vi "Autonomous Independent.vi"() -> ()   [LabVIEW 2014]
doc: "This VI is called when autonomous begins, and will automatically be terminated when autonomous ends. You can carry out timed or sensor driven robot movement independently without needing to return to the caller."
uses:
  <vilib>/Rock Robotics/WPI/Joystick/WPI_JoystickGetSetRefNum.vi
  <vilib>/Rock Robotics/Network Tables/SD Read Number.vi
  <vilib>/Rock Robotics/Network Tables/SD Write String.vi
  <vilib>/Rock Robotics/WPI/RobotDrive/WPI_RobotDriveGetSetRefNum.vi
  <vilib>/Rock Robotics/WPI/RobotDrive/WPI_RobotDriveArcadeDrive_Standard(NoSaturation).vi
panel:
  out "Current Movement, for debugging":T1 {"Y Joystick Value" scale=1.0..-1.0; "X Joystick Value" scale=-1.0..1.0}
  in  "Array of robot movements":T2(array[cluster]) {"Y Joystick Value" scale=1.0..-1.0; "X Joystick Value" scale=-1.0..1.0}
  # "Be sure to right-click and choose Data Operations>>Make Current Value default if you want to save the array values with the VI"
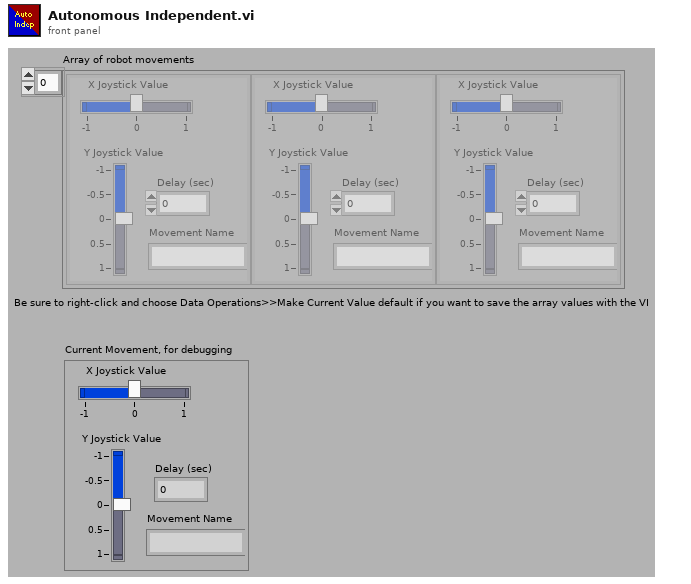
[diagram p1: front panel]
types:
  T1 = cluster{"X Joystick Value":dbl, "Y Joystick Value":dbl, "Delay (sec)":dbl, "Movement Name":string}
  T2 = cluster{"X Joystick Value":dbl, "Y Joystick Value":dbl, "Delay (sec)":dbl, "Movement Name":string}[]
  T3 = typedef "WPI_JoystickDevRef.ctl" = cluster{"Device":T4}
  T4 = typedef "WPI_JoystickDeviceEnum.ctl" = enum16{"USB 0", "USB 1", "USB 2", "USB 3", "USB 4", "USB 5"}
  T5 = typedef "WPI_RobotDriveDevRef.ctl" = cluster{"DevStatus":errorcluster, "Motors[]":T6[], "Square Inputs":bool, "Max Output":dbl}
  T6 = typedef "WPI_MotorControlDeviceRef.ctl" = cluster{"DeviceStatus":errorcluster, "Type":T7, "PWM":cluster{"Controller":T8, "PWM Channel":T9, "DeadBand":T10}, "CAN":cluster{"Device Number":u8, "Control Mode":T11, "Semaphore":T12, "Max Vout":dbl, "TalonSRX Control Mode":T13}, "Invert":bool, "TransformRef":T14, "InvTransformRef":T14}
  T7 = typedef "WPI_MotorControlType.ctl" = enum16{"PWM", "CAN", "CANTalonSRX"}
  T8 = typedef "FPGA_TypedefDigitalModule.ctl" = enum16{"Controller 1"}
  T9 = typedef "FPGA_DIOPWMChannel.ctl" = enum8{"PWM 0", "PWM 1", "PWM 2", "PWM 3", "PWM 4", "PWM 5", "PWM 6", "PWM 7", "PWM 8", "PWM 9", "PWM MXP 0", "PWM MXP 1", "PWM MXP 2", "PWM MXP 3", "PWM MXP 4", "PWM MXP 5", "PWM MXP 6", "PWM MXP 7", "PWM MXP 8", "PWM MXP 9", "Invalid"}
  T10 = typedef "WPI_PWMDeadband.ctl" = cluster{"Name":string, "maxPositivePwm":i32, "minPositivePwm":i32, "centerPwm":i32, "maxNegativePwm":i32, "minNegativePwm":i32, "angularRange":u16}
  T11 = typedef "WPI_CANJaguar_ControlMode.ctl" = enum8{"Percent VBus", "Current", "Speed", "Position", "Voltage"}
  T12 = typedef "Semaphore RefNum" = refnum<k1>
  T13 = typedef "WPI_CANTalonSRX_APIControlMode.ctl" = enum8{"Percent VBus", "Speed", "Position", "Slave", "Unchanged / Invalid"}
  T14 = typedef "WPI_PWMTransform_ConPane.ctl" = refnum<vi>
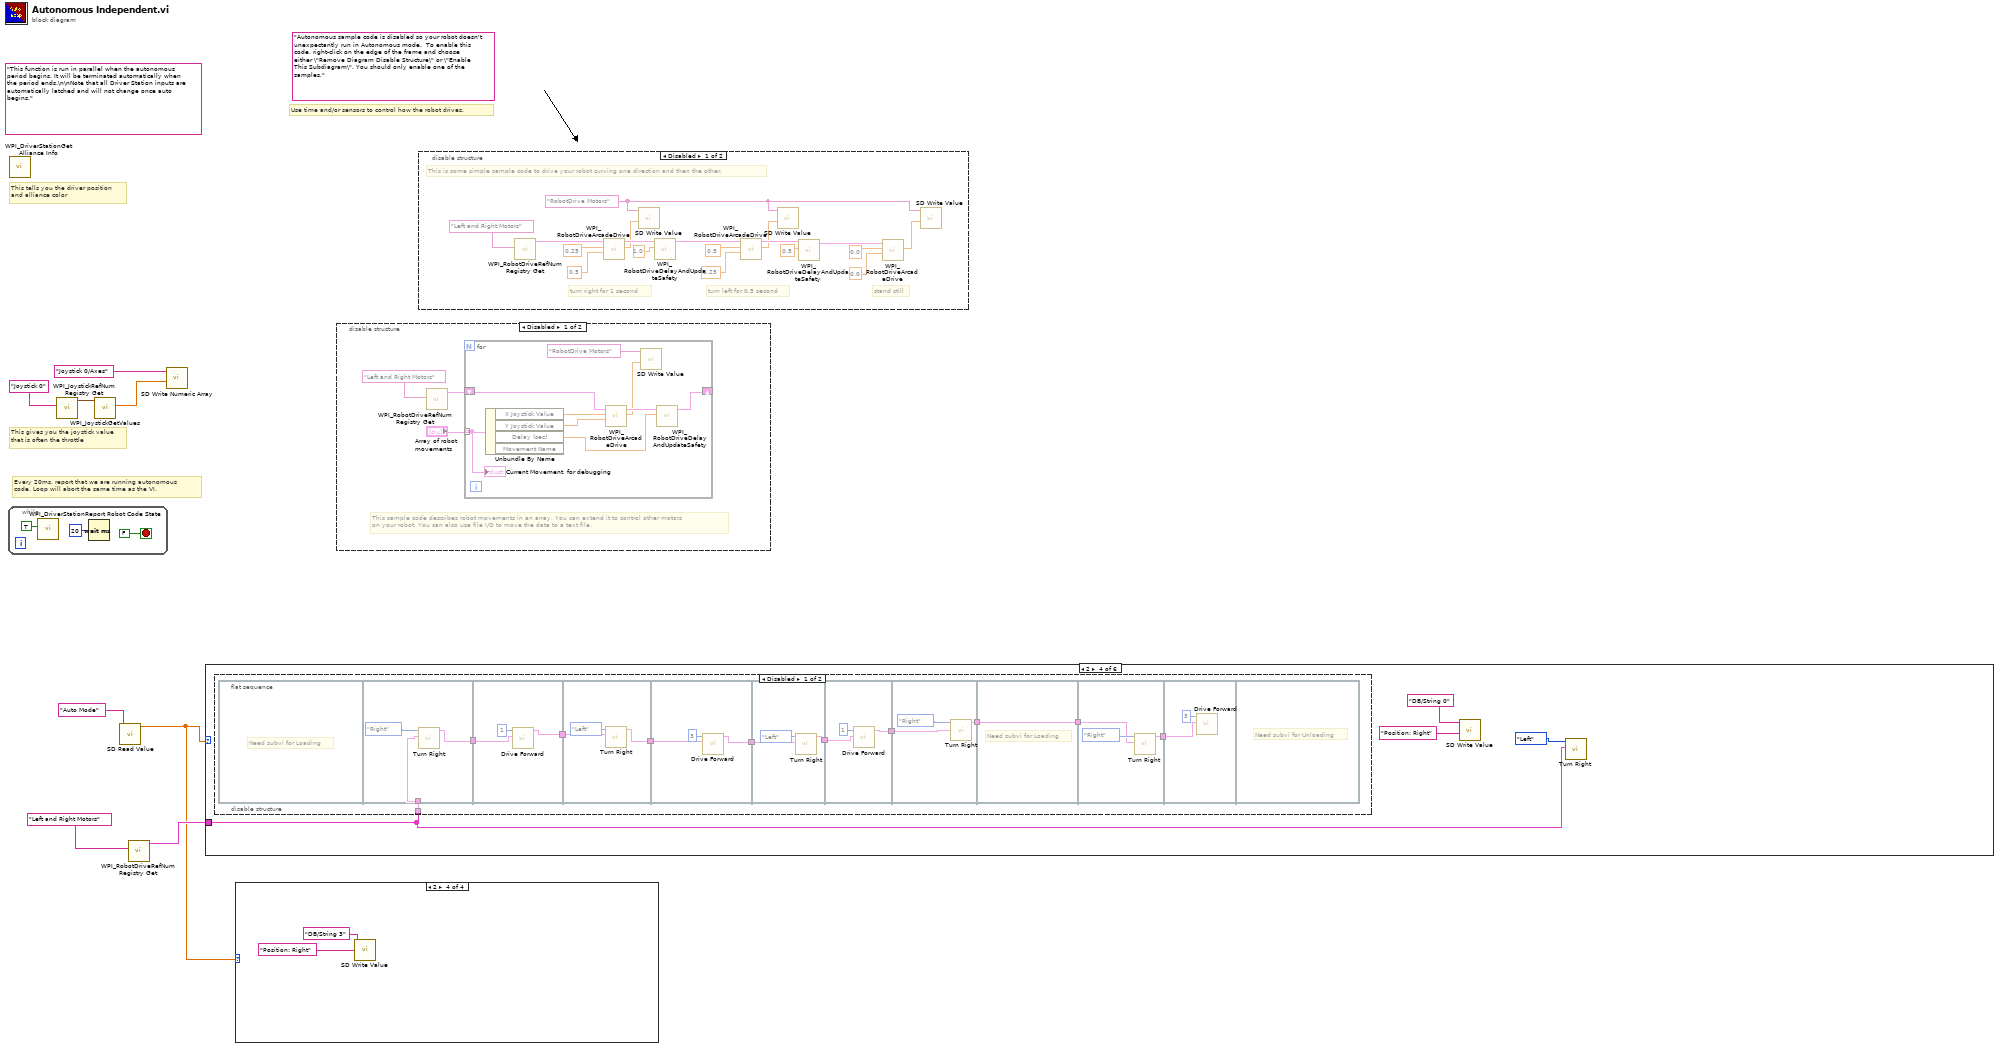
[diagram p0: block diagram]
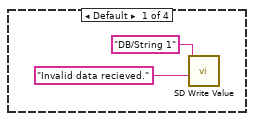
[diagram p2: hidden frame]
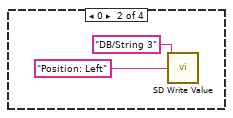
[diagram p3: hidden frame]
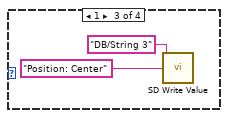
[diagram p4: hidden frame]
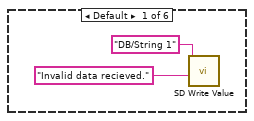
[diagram p5: hidden frame]
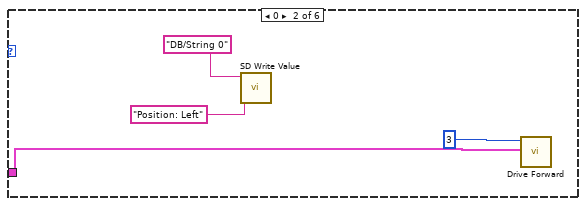
[diagram p6: hidden frame]
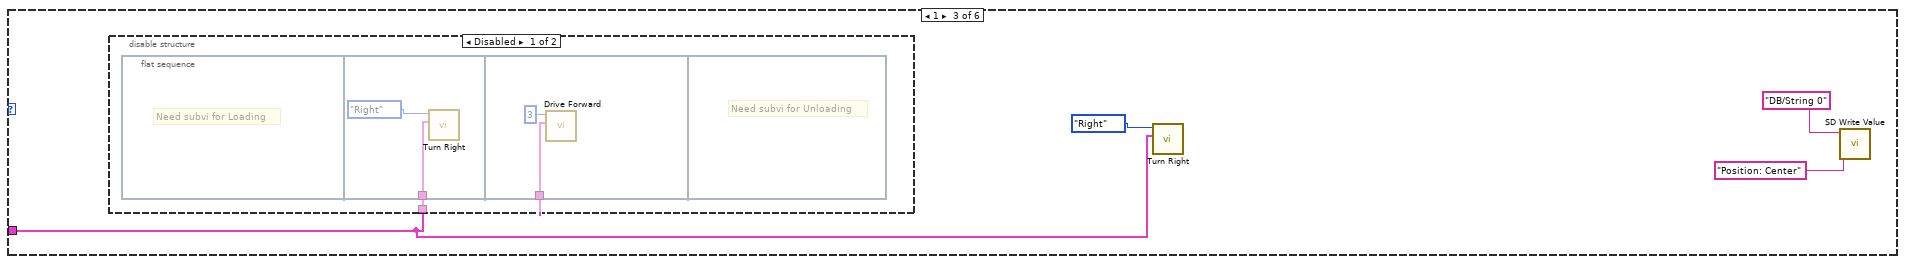
[diagram p7: hidden frame]
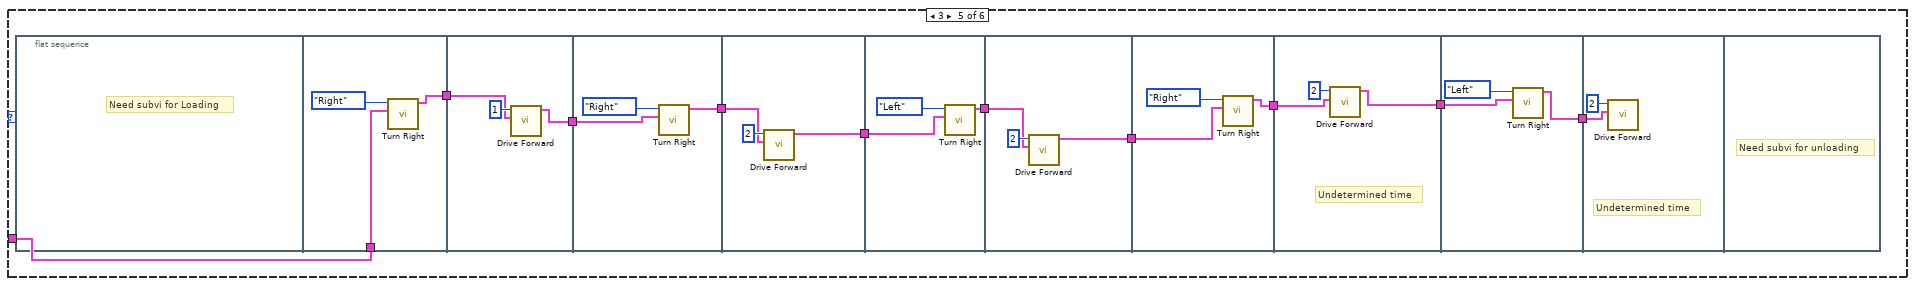
[diagram p10: hidden frame]
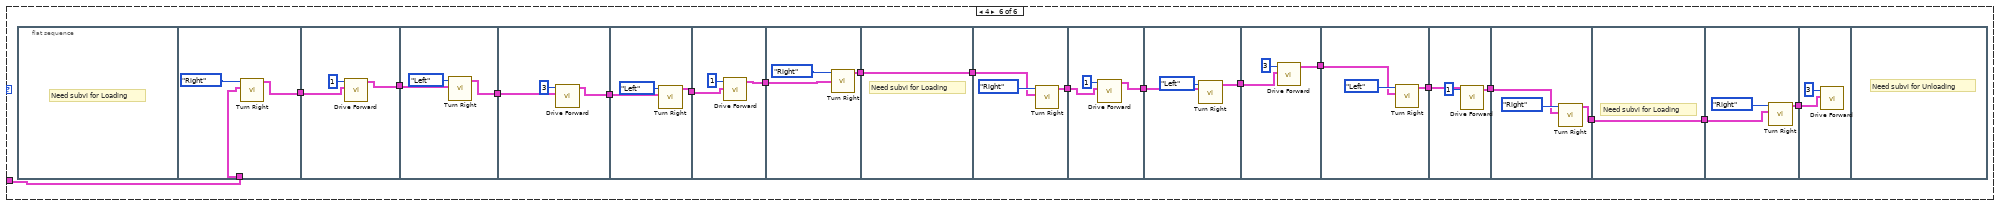
[diagram p11: hidden frame]
diagram:
  (unwired) "Autonomous sample code is disabled so your robot doesn't unexpectantly run in Autonomous mode.  To enable this code, right-click on the edge of the frame and choose either \"Remove Diagram Disable Structure\" or \"Enable This Subdiagram\". You should only enable one of the samples."
  (unwired) "This function is run in parallel when the autonomous period begins. It will be terminated automatically when the period ends.\n\nNote that all Driver Station inputs are automatically latched and will not change once auto begins."
  # "Every 20ms, report that we are running autonomous\ncode. Loop will abort the same time as the VI."
  # "This gives you the joystick value\nthat is often the throttle"
  # "Use time and/or sensors to control how the robot drives."
  # "This tells you the driver position\nand alliance color"
  n1 = while {
    stop <- FALSE stop-if-true
    n2 = call <vilib>:"WPI_DriverStationReport Robot Code State.vi"("Autonomous"=TRUE) -> ()  [unwired: 10 in, 1 out]
    n3 = Wait (ms)(milliseconds to wait=u32 20) -> ()  [unwired: 1 out]
  }
  n4 = call <vilib>:"WPI_DriverStationGet Alliance Info.vi"() -> ()  [unwired: 12 out]
  n5 = call <vilib>:"WPI_JoystickRefNum Registry Get.vi"("refnum name"="Joystick 0") -> ("JoystickDevRef"=w7:T3)  [unwired: 1 in, 9 out]
  n6 = call <vilib>:"WPI_JoystickGetValues.vi"("JoystickDevRef"=w7) -> ("Axes"=w5:dbl[])  [unwired: 6 in, 4 out]
  n7 = call-poly <vilib>:"SD Read Value.vi"("Name"="Auto Mode") -> ("Numeric"=w1:dbl)  [unwired: 8 in, 2 out]
  n8 = call <vilib>:"WPI_RobotDriveRefNum Registry Get.vi"("refnum name"="Left and Right Motors") -> ("RobotDriveDevRef"=w2:T5)  [unwired: 9 in, 1 out]
  n9 = call <vilib>:"SD Write Numeric Array.vi"("Numeric Array"=w5, "Name"="Joystick 0/Axes") -> ()  [unwired: 8 in, 2 out]
  n10 = case shown="2" w1 {
    tunnel: w2 -> [_ w14 w18 w27 w77 w116]
    frame Default {
      n11 = call-poly <vilib>:"SD Write Value.vi"("String"="Invalid data recieved.", "Name"="DB/String 1") -> ()  [unwired: 8 in, 2 out]
    }
    frame 0 {
      n12 = call-poly <vilib>:"SD Write Value.vi"("String"="Position: Left", "Name"="DB/String 0") -> ()  [unwired: 8 in, 2 out]
      n13 = call "Drive Forward.vi"("RobotDriveDevRef in"=w14, "Numeric"=3) -> ()  [unwired: 9 in, 1 out]
    }
    frame 1 {
      n14 = disable-structure shown="Disabled" {
        disable-tunnel: w18 -> [w22 _]
        frame Disabled {
          n15 = flat-sequence {
            tunnel: w22 -> [w23]
            tunnel: w22 -> [w25]
            frame #0 {
              # "Need subvi for Loading"
            }
            frame #1 {
              n16 = call "Turn Right.vi"("RobotDriveDevRef in"=w23, "Turn Direction"=enum16{"Right", "Left"}."Right") -> ()  [unwired: 9 in, 1 out]
            }
            frame #2 {
              n17 = call "Drive Forward.vi"("RobotDriveDevRef in"=w25, "Numeric"=3) -> ()  [unwired: 9 in, 1 out]
            }
            frame #3 {
              # "Need subvi for Unloading"
            }
          }
        }
        frame Enabled {
        }
      }
      n18 = call "Turn Right.vi"("RobotDriveDevRef in"=w18, "Turn Direction"=enum16{"Right", "Left"}."Right") -> ()  [unwired: 9 in, 1 out]
      n19 = call-poly <vilib>:"SD Write Value.vi"("String"="Position: Center", "Name"="DB/String 0") -> ()  [unwired: 8 in, 2 out]
    }
    frame 2 {
      n20 = disable-structure shown="Disabled" {
        disable-tunnel: w27 -> [w31 _]
        frame Disabled {
          n21 = flat-sequence {
            tunnel: w31 -> [w42]
            tunnel: [w41] -> w40
            tunnel: w40 -> [w45]
            tunnel: [w44] -> w39
            tunnel: w39 -> [w49]
            tunnel: [w47] -> w38
            tunnel: w38 -> [w52]
            tunnel: [w50] -> w37
            tunnel: w37 -> [w54]
            tunnel: [w53] -> w36
            tunnel: w36 -> [w57]
            tunnel: [w56] -> w35
            tunnel: w35 -> [w60]
            tunnel: [w59] -> w34
            tunnel: [w62] -> w33
            tunnel: w34 -> [w62]
            tunnel: w33 -> [w64]
            tunnel: [w63] -> w32
            tunnel: w32 -> [w66]
            frame #0 {
              # "Need subvi for Loading"
            }
            frame #1 {
              n22 = call "Turn Right.vi"("RobotDriveDevRef in"=w42, "Turn Direction"=enum16{"Right", "Left"}."Right") -> ("RobotDriveDevRef out"=w41:T5)  [unwired: 9 in]
            }
            frame #2 {
              n23 = call "Drive Forward.vi"("RobotDriveDevRef in"=w45, "Numeric"=1) -> ("RobotDriveDevRef out"=w44:T5)  [unwired: 9 in]
            }
            frame #3 {
              n24 = call "Turn Right.vi"("RobotDriveDevRef in"=w49, "Turn Direction"=enum16{"Right", "Left"}."Left") -> ("RobotDriveDevRef out"=w47:T5)  [unwired: 9 in]
            }
            frame #4 {
              n25 = call "Drive Forward.vi"("RobotDriveDevRef in"=w52, "Numeric"=3) -> ("RobotDriveDevRef out"=w50:T5)  [unwired: 9 in]
            }
            frame #5 {
              n26 = call "Turn Right.vi"("RobotDriveDevRef in"=w54, "Turn Direction"=enum16{"Right", "Left"}."Left") -> ("RobotDriveDevRef out"=w53:T5)  [unwired: 9 in]
            }
            frame #6 {
              n27 = call "Drive Forward.vi"("RobotDriveDevRef in"=w57, "Numeric"=1) -> ("RobotDriveDevRef out"=w56:T5)  [unwired: 9 in]
            }
            frame #7 {
              n28 = call "Turn Right.vi"("RobotDriveDevRef in"=w60, "Turn Direction"=enum16{"Right", "Left"}."Right") -> ("RobotDriveDevRef out"=w59:T5)  [unwired: 9 in]
            }
            frame #8 {
              # "Need subvi for Loading"
            }
            frame #9 {
              n29 = call "Turn Right.vi"("RobotDriveDevRef in"=w64, "Turn Direction"=enum16{"Right", "Left"}."Right") -> ("RobotDriveDevRef out"=w63:T5)  [unwired: 9 in]
            }
            frame #10 {
              n30 = call "Drive Forward.vi"("RobotDriveDevRef in"=w66, "Numeric"=3) -> ()  [unwired: 9 in, 1 out]
            }
            frame #11 {
              # "Need subvi for Unloading"
            }
          }
        }
        frame Enabled {
        }
      }
      n31 = call-poly <vilib>:"SD Write Value.vi"("String"="Position: Right", "Name"="DB/String 0") -> ()  [unwired: 8 in, 2 out]
      n32 = call "Turn Right.vi"("RobotDriveDevRef in"=w27, "Turn Direction"=enum16{"Right", "Left"}."Left") -> ()  [unwired: 9 in, 1 out]
    }
    frame 3 {
      n33 = flat-sequence {
        tunnel: w77 -> [w79]
        tunnel: [w78] -> w76
        tunnel: w76 -> [w82]
        tunnel: [w81] -> w75
        tunnel: w75 -> [w85]
        tunnel: [w84] -> w74
        tunnel: w74 -> [w88]
        tunnel: [w87] -> w73
        tunnel: w73 -> [w91]
        tunnel: [w90] -> w72
        tunnel: w72 -> [w94]
        tunnel: [w93] -> w71
        tunnel: w71 -> [w97]
        tunnel: [w96] -> w70
        tunnel: w70 -> [w100]
        tunnel: [w99] -> w69
        tunnel: w69 -> [w103]
        tunnel: [w102] -> w68
        tunnel: w68 -> [w105]
        frame #0 {
          # "Need subvi for Loading"
        }
        frame #1 {
          n34 = call "Turn Right.vi"("RobotDriveDevRef in"=w79, "Turn Direction"=enum16{"Right", "Left"}."Right") -> ("RobotDriveDevRef out"=w78:T5)  [unwired: 9 in]
        }
        frame #2 {
          n35 = call "Drive Forward.vi"("RobotDriveDevRef in"=w82, "Numeric"=1) -> ("RobotDriveDevRef out"=w81:T5)  [unwired: 9 in]
        }
        frame #3 {
          n36 = call "Turn Right.vi"("RobotDriveDevRef in"=w85, "Turn Direction"=enum16{"Right", "Left"}."Right") -> ("RobotDriveDevRef out"=w84:T5)  [unwired: 9 in]
        }
        frame #4 {
          n37 = call "Drive Forward.vi"("RobotDriveDevRef in"=w88, "Numeric"=2) -> ("RobotDriveDevRef out"=w87:T5)  [unwired: 9 in]
        }
        frame #5 {
          n38 = call "Turn Right.vi"("RobotDriveDevRef in"=w91, "Turn Direction"=enum16{"Right", "Left"}."Left") -> ("RobotDriveDevRef out"=w90:T5)  [unwired: 9 in]
        }
        frame #6 {
          n39 = call "Drive Forward.vi"("RobotDriveDevRef in"=w94, "Numeric"=2) -> ("RobotDriveDevRef out"=w93:T5)  [unwired: 9 in]
        }
        frame #7 {
          n40 = call "Turn Right.vi"("RobotDriveDevRef in"=w97, "Turn Direction"=enum16{"Right", "Left"}."Right") -> ("RobotDriveDevRef out"=w96:T5)  [unwired: 9 in]
        }
        frame #8 {
          # "Undetermined time"
          n41 = call "Drive Forward.vi"("RobotDriveDevRef in"=w100, "Numeric"=2) -> ("RobotDriveDevRef out"=w99:T5)  [unwired: 9 in]
        }
        frame #9 {
          n42 = call "Turn Right.vi"("RobotDriveDevRef in"=w103, "Turn Direction"=enum16{"Right", "Left"}."Left") -> ("RobotDriveDevRef out"=w102:T5)  [unwired: 9 in]
        }
        frame #10 {
          # "Undetermined time"
          n43 = call "Drive Forward.vi"("RobotDriveDevRef in"=w105, "Numeric"=2) -> ()  [unwired: 9 in, 1 out]
        }
        frame #11 {
          # "Need subvi for unloading"
        }
      }
    }
    frame 4 {
      n44 = flat-sequence {
        tunnel: w116 -> [w126]
        tunnel: [w125] -> w124
        tunnel: w124 -> [w129]
        tunnel: [w128] -> w123
        tunnel: w123 -> [w133]
        tunnel: [w131] -> w122
        tunnel: w122 -> [w136]
        tunnel: [w134] -> w121
        tunnel: w121 -> [w138]
        tunnel: [w137] -> w120
        tunnel: w120 -> [w141]
        tunnel: [w140] -> w119
        tunnel: w119 -> [w144]
        tunnel: [w143] -> w118
        tunnel: [w146] -> w117
        tunnel: w118 -> [w146]
        tunnel: w117 -> [w148]
        tunnel: [w147] -> w115
        tunnel: w115 -> [w151]
        tunnel: [w150] -> w114
        tunnel: w114 -> [w154]
        tunnel: [w153] -> w113
        tunnel: w113 -> [w157]
        tunnel: [w156] -> w112
        tunnel: w112 -> [w160]
        tunnel: [w159] -> w111
        tunnel: w111 -> [w163]
        tunnel: [w162] -> w110
        tunnel: w110 -> [w166]
        tunnel: [w165] -> w108
        tunnel: [w168] -> w109
        tunnel: w108 -> [w168]
        tunnel: w109 -> [w170]
        tunnel: [w169] -> w107
        tunnel: w107 -> [w172]
        frame #0 {
          # "Need subvi for Loading"
        }
        frame #1 {
          n45 = call "Turn Right.vi"("RobotDriveDevRef in"=w126, "Turn Direction"=enum16{"Right", "Left"}."Right") -> ("RobotDriveDevRef out"=w125:T5)  [unwired: 9 in]
        }
        frame #2 {
          n46 = call "Drive Forward.vi"("RobotDriveDevRef in"=w129, "Numeric"=1) -> ("RobotDriveDevRef out"=w128:T5)  [unwired: 9 in]
        }
        frame #3 {
          n47 = call "Turn Right.vi"("RobotDriveDevRef in"=w133, "Turn Direction"=enum16{"Right", "Left"}."Left") -> ("RobotDriveDevRef out"=w131:T5)  [unwired: 9 in]
        }
        frame #4 {
          n48 = call "Drive Forward.vi"("RobotDriveDevRef in"=w136, "Numeric"=3) -> ("RobotDriveDevRef out"=w134:T5)  [unwired: 9 in]
        }
        frame #5 {
          n49 = call "Turn Right.vi"("RobotDriveDevRef in"=w138, "Turn Direction"=enum16{"Right", "Left"}."Left") -> ("RobotDriveDevRef out"=w137:T5)  [unwired: 9 in]
        }
        frame #6 {
          n50 = call "Drive Forward.vi"("RobotDriveDevRef in"=w141, "Numeric"=1) -> ("RobotDriveDevRef out"=w140:T5)  [unwired: 9 in]
        }
        frame #7 {
          n51 = call "Turn Right.vi"("RobotDriveDevRef in"=w144, "Turn Direction"=enum16{"Right", "Left"}."Right") -> ("RobotDriveDevRef out"=w143:T5)  [unwired: 9 in]
        }
        frame #8 {
          # "Need subvi for Loading"
        }
        frame #9 {
          n52 = call "Turn Right.vi"("RobotDriveDevRef in"=w148, "Turn Direction"=enum16{"Right", "Left"}."Right") -> ("RobotDriveDevRef out"=w147:T5)  [unwired: 9 in]
        }
        frame #10 {
          n53 = call "Drive Forward.vi"("RobotDriveDevRef in"=w151, "Numeric"=1) -> ("RobotDriveDevRef out"=w150:T5)  [unwired: 9 in]
        }
        frame #11 {
          n54 = call "Turn Right.vi"("RobotDriveDevRef in"=w154, "Turn Direction"=enum16{"Right", "Left"}."Left") -> ("RobotDriveDevRef out"=w153:T5)  [unwired: 9 in]
        }
        frame #12 {
          n55 = call "Drive Forward.vi"("RobotDriveDevRef in"=w157, "Numeric"=3) -> ("RobotDriveDevRef out"=w156:T5)  [unwired: 9 in]
        }
        frame #13 {
          n56 = call "Turn Right.vi"("RobotDriveDevRef in"=w160, "Turn Direction"=enum16{"Right", "Left"}."Left") -> ("RobotDriveDevRef out"=w159:T5)  [unwired: 9 in]
        }
        frame #14 {
          n57 = call "Drive Forward.vi"("RobotDriveDevRef in"=w163, "Numeric"=1) -> ("RobotDriveDevRef out"=w162:T5)  [unwired: 9 in]
        }
        frame #15 {
          n58 = call "Turn Right.vi"("RobotDriveDevRef in"=w166, "Turn Direction"=enum16{"Right", "Left"}."Right") -> ("RobotDriveDevRef out"=w165:T5)  [unwired: 9 in]
        }
        frame #16 {
          # "Need subvi for Loading"
        }
        frame #17 {
          n59 = call "Turn Right.vi"("RobotDriveDevRef in"=w170, "Turn Direction"=enum16{"Right", "Left"}."Right") -> ("RobotDriveDevRef out"=w169:T5)  [unwired: 9 in]
        }
        frame #18 {
          n60 = call "Drive Forward.vi"("RobotDriveDevRef in"=w172, "Numeric"=3) -> ()  [unwired: 9 in, 1 out]
        }
        frame #19 {
          # "Need subvi for Unloading"
        }
      }
    }
  }
  n61 = case shown="2" w1 {
    frame Default {
      n62 = call-poly <vilib>:"SD Write Value.vi"("String"="Invalid data recieved.", "Name"="DB/String 1") -> ()  [unwired: 8 in, 2 out]
    }
    frame 0 {
      n63 = call-poly <vilib>:"SD Write Value.vi"("String"="Position: Left", "Name"="DB/String 3") -> ()  [unwired: 8 in, 2 out]
    }
    frame 1 {
      n64 = call-poly <vilib>:"SD Write Value.vi"("String"="Position: Center", "Name"="DB/String 3") -> ()  [unwired: 8 in, 2 out]
    }
    frame 2 {
      n65 = call-poly <vilib>:"SD Write Value.vi"("String"="Position: Right", "Name"="DB/String 3") -> ()  [unwired: 8 in, 2 out]
    }
  }
  n66 = disable-structure shown="Disabled" {
    frame Disabled {
      # "This sample code describes robot movements in an array. You can extend it to control other motors\non your robot. You can also use file I/O to move the data to a text file."
      n67 = call <vilib>:"WPI_RobotDriveRefNum Registry Get.vi"("refnum name"="Left and Right Motors") -> ("RobotDriveDevRef"=w183:T5)  [unwired: 1 in, 9 out]
      n68 = for {
        shift-right: [w190] -> _
        shift-left: w183 -> [w191]
        tunnel: "Array of robot movements" -> [w186] mode=indexing
        n69 = Unbundle By Name(w186) -> ("X Joystick Value"=w189:dbl, "Y Joystick Value"=w188:dbl, "Delay (sec)"=w187:dbl)  [unwired: 1 out]
        n70 = call-poly <vilib>:"WPI_RobotDriveArcadeDrive.vi"("Y axis value"=w188, "X axis value"=w189, "RobotDriveDevRef"=w191) -> ("Motor Values"=w185:dbl[], "RobotDriveDevRef"=w192:T5)  [unwired: 1 in, 6 out]
        n71 = call-poly <vilib>:"SD Write Value.vi"("Numeric Array"=w185, "Name"="RobotDrive Motors") -> ()  [unwired: 8 in, 2 out]
        n72 = call <vilib>:"WPI_RobotDriveDelayAndUpdateSafety.vi"("Delay (s)"=w187, "RobotDriveDevRef"=w192) -> ("RobotDriveDevRef 2"=w190:T5)  [unwired: 8 in, 1 out]
        "Current Movement, for debugging" <- w186
      }
    }
    frame Enabled {
    }
  }
  n73 = disable-structure shown="Disabled" {
    frame Disabled {
      w197 = "RobotDrive Motors" ("Name")
      # "This is some simple sample code to drive your robot curving one direction and then the other."
      # "stand still"
      # "turn left for 0.5 second"
      # "turn right for 1 second"
      n74 = call <vilib>:"WPI_RobotDriveRefNum Registry Get.vi"("refnum name"="Left and Right Motors") -> ("RobotDriveDevRef"=w198:T5)  [unwired: 1 in, 9 out]
      n75 = call-poly <vilib>:"WPI_RobotDriveArcadeDrive.vi"("Y axis value"=0.5 ("X axis value"), "X axis value"=0.25, "RobotDriveDevRef"=w198) -> ("Motor Values"=w196:dbl[], "RobotDriveDevRef"=w205:T5)  [unwired: 1 in, 6 out]
      n76 = call-poly <vilib>:"SD Write Value.vi"("Numeric Array"=w196, "Name"=w197) -> ()  [unwired: 8 in, 2 out]
      n77 = call <vilib>:"WPI_RobotDriveDelayAndUpdateSafety.vi"("Delay (s)"=1.0, "RobotDriveDevRef"=w205) -> ("RobotDriveDevRef 2"=w204:T5)  [unwired: 8 in, 1 out]
      n78 = call-poly <vilib>:"WPI_RobotDriveArcadeDrive.vi"("Y axis value"=0.25 ("X axis value"), "X axis value"=0.5, "RobotDriveDevRef"=w204) -> ("Motor Values"=w195:dbl[], "RobotDriveDevRef"=w203:T5)  [unwired: 1 in, 6 out]
      n79 = call-poly <vilib>:"SD Write Value.vi"("Numeric Array"=w195, "Name"=w197) -> ()  [unwired: 8 in, 2 out]
      n80 = call <vilib>:"WPI_RobotDriveDelayAndUpdateSafety.vi"("Delay (s)"=0.5, "RobotDriveDevRef"=w203) -> ("RobotDriveDevRef 2"=w202:T5)  [unwired: 8 in, 1 out]
      n81 = call-poly <vilib>:"WPI_RobotDriveArcadeDrive.vi"("Y axis value"=0.0 ("X axis value"), "X axis value"=0.0, "RobotDriveDevRef"=w202) -> ("Motor Values"=w194:dbl[])  [unwired: 1 in, 7 out]
      n82 = call-poly <vilib>:"SD Write Value.vi"("Numeric Array"=w194, "Name"=w197) -> ()  [unwired: 8 in, 2 out]
    }
    frame Enabled {
    }
  }
